vi "Tree Set Symbol.vi"(8 "error in (no error)":errorcluster, 11 "Tree in":refnum<vi>) -> (0 "error out":errorcluster, 3 "Tree out":refnum<vi>)   [LabVIEW 2017]
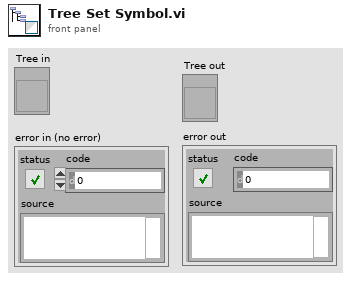
[diagram p1: front panel]
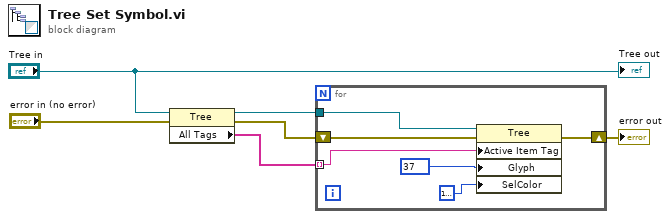
[diagram p0: block diagram]
diagram:
  n1 = property on="Property Node" class="Tree"(reference="Tree in", error in="error in (no error)") -> (reference out=w4:refnum<vi>, error out=w3:errorcluster, "All Tags"=w5:string[])
  n2 = for {
    shift-right: [w11] -> w6
    shift-left: w3 -> [w10]
    tunnel: w5 -> [w9] mode=indexing
    tunnel: w4 -> [w8]
    n3 = property class="Tree"(reference=w8, error in=w10, "Active Item Tag"=w9, "Glyph"=37, "SelColor"=u32 16777216) -> (error out=w11:errorcluster)  [unwired: 1 out]
  }
  "error out" <- w6
  "Tree out" <- "Tree in"
